vi "cal_c_theta.vi"(2 "£c":dbl, 3 "c":dbl, 4 "b":dbl, 5 "a":dbl) -> (0 "theta":dbl, 1 "c":dbl)   [LabVIEW 2019]
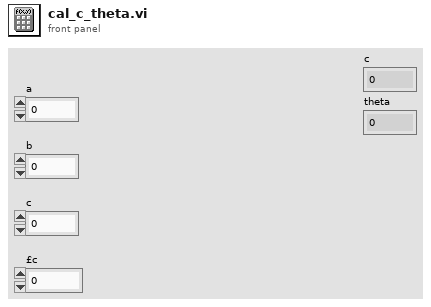
[diagram p1: front panel]
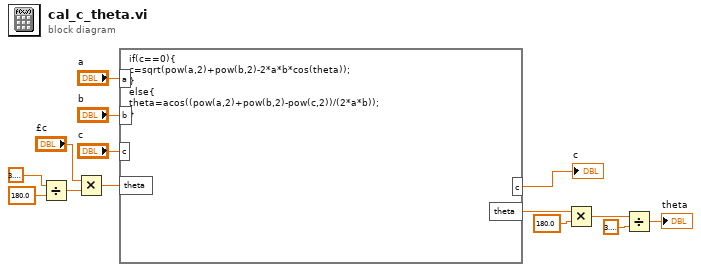
[diagram p0: block diagram]
diagram:
  n1 = Divide(x=3.141592653589793, y=180.0 ("x")) -> (x/y=w8:dbl)
  n2 = Multiply(x="£c", y=w8) -> (x*y=w7:dbl)
  n3 = formula code="if(c==0){\nc=sqrt(pow(a,2)+pow(b,2)-2*a*b*cos(theta));\n}\nelse{\ntheta=acos((pow(a,2)+pow(b,2)-pow(c,2))/(2*a*b));\n}"("a"="a", "b"="b", "c"="c", "theta"=w7) -> ("c"=→"c":dbl, "theta"=w5:dbl)
  n4 = Multiply(x=w5, y=180.0) -> (x*y=w3:dbl)
  n5 = Divide(x=w3, y=3.141592653589793) -> (x/y=→"theta":dbl)
